vi "Motor Command.vi"(8 "error in (no error)":errorcluster, 11 "output cluster":T1) -> (0 "error out":errorcluster)   [LabVIEW 2016]
uses:
  Que Cluster TD.ctl
  Que Attributes TD.ctl
  Que enum td.ctl
  <vilib>/addons/zeromq/socket_type.ctl
  <vilib>/addons/zeromq/socket_options.ctl
  <vilib>/addons/zeromq/zeromq.lvlib
  <vilib>/addons/zeromq/zmq_context.lvclass
  <vilib>/addons/zeromq/zmq_socket.lvclass
panel:
  out "data":string
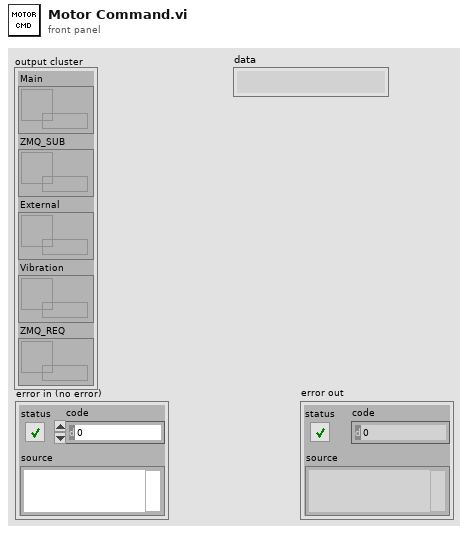
[diagram p1: front panel]
types:
  T1 = typedef "Que Cluster TD.ctl" = cluster{"Main":refnum<queue>, "ZMQ_SUB":refnum<queue>, "External":refnum<queue>, "Vibration":refnum<queue>, "ZMQ_REQ":refnum<queue>}
  T2 = typedef "zeromq.lvlib/socket_options.ctl" = enum8{"NONE", "ZMQ_HWM", "<2>", "ZMQ_SWAP", "ZMQ_AFFINITY", "ZMQ_IDENTITY", "ZMQ_SUBSCRIBE", "ZMQ_UNSUBSCRIBE", "ZMQ_RATE", "ZMQ_RECOVERY_IVL", "ZMQ_MCAST_LOOP", "ZMQ_SNDBUF", "ZMQ_RCVBUF", "ZMQ_RCVMORE", "ZMQ_FD", "ZMQ_EVENTS", "ZMQ_TYPE", "ZMQ_LINGER", "ZMQ_RECONNECT_IVL", "ZMQ_BACKLOG", "ZMQ_RECOVERY_IVL_MSEC", "ZMQ_RECONNECT_IVL_MAX", "ZMQ_MAXMSGSIZE", "ZMQ_SNDHWM", "ZMQ_RCVHWM", "ZMQ_MULTICAST_HOPS", "<26>", "ZMQ_RCVTIMEO", "ZMQ_SNDTIMEO", "<29>", "<30>", "ZMQ_IPV4ONLY", "ZMQ_LAST_ENDPOINT", "ZMQ_ROUTER_MANDATORY", "ZMQ_TCP_KEEPALIVE", "ZMQ_TCP_KEEPALIVE_CNT", "ZMQ_TCP_KEEPALIVE_IDLE", "ZMQ_TCP_KEEPALIVE_INTVL", "ZMQ_TCP_ACCEPT_FILTER", "ZMQ_DELAY_ATTACH_ON_CONNECT", "ZMQ_XPUB_VERBOSE"}
  T3 = typedef "zeromq.lvlib/socket_type.ctl" = enum8{"ZMQ_PAIR", "ZMQ_PUB", "ZMQ_SUB", "ZMQ_REQ", "ZMQ_REP", "ZMQ_DEALER", "ZMQ_ROUTER", "ZMQ_PULL", "ZMQ_PUSH", "ZMQ_XPUB", "ZMQ_XSUB"}
  T4 = typedef "Que Attributes TD.ctl" = cluster{"Que States":T5, "String":string, "Boolean":bool, "Double":dbl, "U16":u16}
  T5 = typedef "Que enum td.ctl" = enum16{"Stop", "Start", "Update D_HW", "Initialize", "Exit", "Read", "Write", "Plot", "Log", "Stop Log", "Start Log", "Wait"}
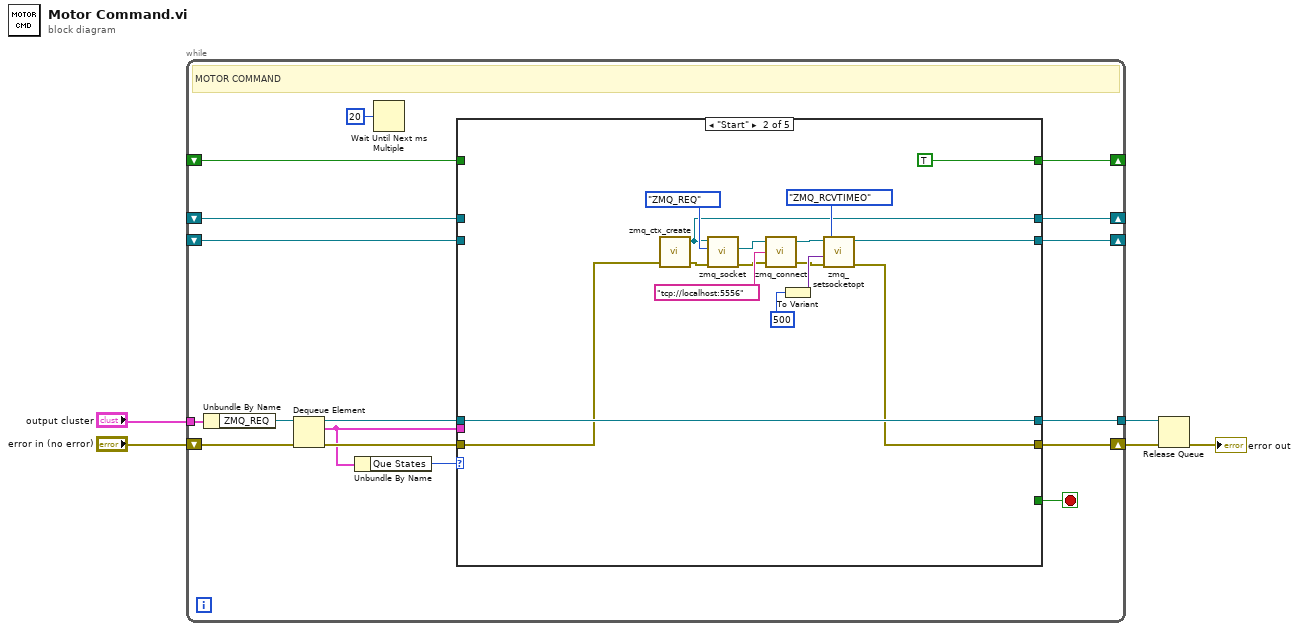
[diagram p0: block diagram]
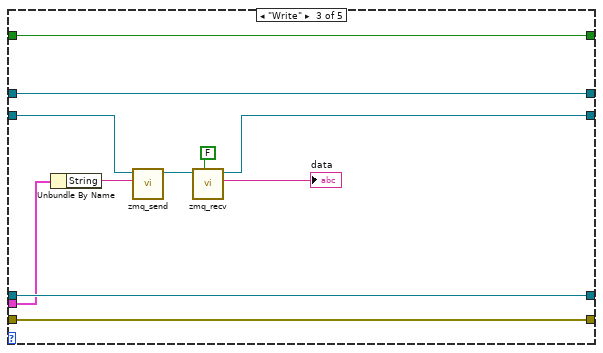
[diagram p3: hidden frame]
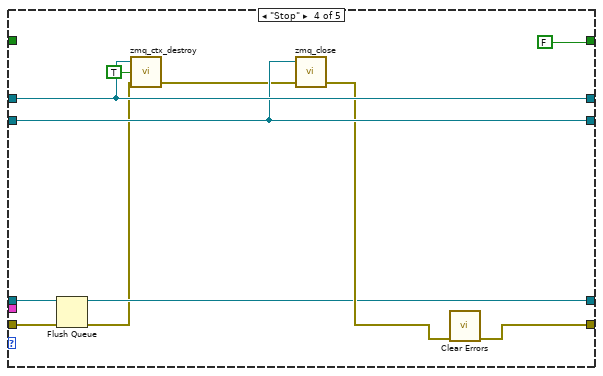
[diagram p4: hidden frame]
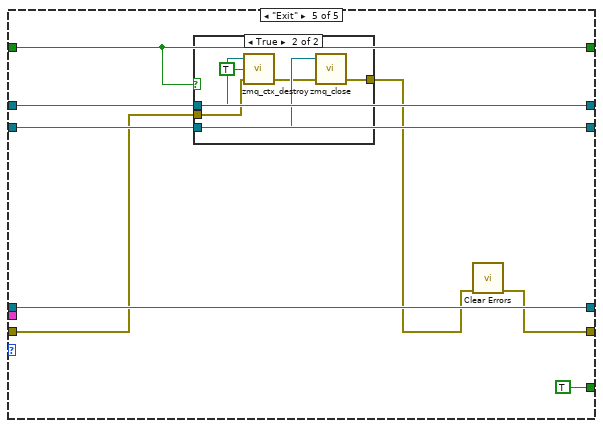
[diagram p5: hidden frame]
diagram:
  n1 = while {
    tunnel: "output cluster" -> [w22]
    tunnel: [w17] -> w4
    shift-right: [w16] -> w5
    shift-left: "error in (no error)" -> [w20]
    shift-right: [w12] -> _
    shift-left: _ -> [w11]
    shift-right: [w9] -> _
    shift-left: _ -> [w8]
    shift-right: [w7] -> _
    shift-left: _ -> [w6]
    stop <- w13 stop-if-true
    # "MOTOR COMMAND"
    n2 = Unbundle By Name(w22) -> ("ZMQ_REQ"=w21:refnum<queue>)
    n3 = Dequeue Element(queue=w21, error in (no error)=w20) -> (queue out=w18:refnum<queue>, element=w10:T4, error out=w19:errorcluster)  [unwired: 1 in, 1 out]
    n4 = Unbundle By Name(w10) -> ("Que States"=w15:T5)
    n5 = Wait Until Next ms Multiple(millisecond multiple=u32 20) -> ()  [unwired: 1 out]
    n6 = case shown="\"Start\"" w15 {
      tunnel: w19 -> [w26 w42 w47 w57 w68]
      tunnel: w18 -> [w27 w43 w54 w59 w73]
      tunnel: [w27 w43 w54 w58 w73] -> w17
      tunnel: [w26 w41 w47 w61 w66] -> w16
      tunnel: [_ _ _ _ TRUE] -> w13
      tunnel: [w25 w40 w50 w64 w70] -> w12
      tunnel: w11 -> [w25 _ w51 w64 w70]
      tunnel: w10 -> [_ _ w49 _ _]
      tunnel: [w24 w29 w45 w65 w71] -> w9
      tunnel: w8 -> [w24 _ w45 w65 w71]
      tunnel: [w23 TRUE w44 FALSE w69] -> w7
      tunnel: w6 -> [w23 _ w44 _ w69]
      frame "Initialize", Default {
      }
      frame "Start" {
        n7 = call <vilib>:"zmq_ctx_create.vi"("error in"=w42) -> ("error out"=w33:errorcluster, "context out"=w29:refnum<class "zmq_context.lvclass">)  [unwired: 3 in]
        n8 = call <vilib>:"zmq_socket.vi"("error in"=w33, "socket type"=socket_type."ZMQ_REQ", "context in"=w29) -> ("error out"=w30:errorcluster, "socket out"=w31:refnum<class "zmq_socket.lvclass">)  [unwired: 2 in, 1 out]
        n9 = call <vilib>:"zmq_connect.vi"("error in"=w30, "endpoint"="tcp://localhost:5556", "socket in"=w31) -> ("error out"=w36:errorcluster, "socket out"=w35:refnum<class "zmq_socket.lvclass">)  [unwired: 1 in]
        n10 = To Variant(anything=500) -> (Variant=w39:variant)
        n11 = call <vilib>:"zmq_setsocketopt.vi"("error in"=w36, "value"=w39, "option"=socket_options."ZMQ_RCVTIMEO", "socket in"=w35) -> ("error out"=w41:errorcluster, "socket out"=w40:refnum<class "zmq_socket.lvclass">)  [unwired: 2 in]
      }
      frame "Write" {
        n12 = Unbundle By Name(w49) -> ("String"=w48:string)
        n13 = call <vilib>:"zmq_send.vi"("data"=w48, "socket in"=w51) -> ("socket out"=w52:refnum<class "zmq_socket.lvclass">)  [unwired: 5 in, 1 out]
        n14 = call <vilib>:"zmq_recv.vi"("no block? (F)"=FALSE, "socket in"=w52) -> ("data"=→"data":string, "socket out"=w50:refnum<class "zmq_socket.lvclass">)  [unwired: 3 in, 3 out]
      }
      frame "Stop" {
        n15 = Flush Queue(queue=w59, error in (no error)=w57) -> (queue out=w58:refnum<queue>, error out=w56:errorcluster)  [unwired: 1 out]
        n16 = call <vilib>:"zmq_ctx_destroy.vi"("error in"=w56, "reap? (F)"=TRUE, "context in"=w65) -> ("error out"=w63:errorcluster)  [unwired: 2 in]
        n17 = call <vilib>:"zmq_close.vi"("error in"=w63, "socket"=w64) -> ("error out"=w62:errorcluster)  [unwired: 3 in]
        n18 = call <vilib>:"Clear Errors.vi"("error in (no error)"=w62) -> ("error out"=w61:errorcluster)  [unwired: 5 in, 1 out]
      }
      frame "Exit" {
        n19 = case shown="True" w69 {
          tunnel: w71 -> [_ w80]
          tunnel: w70 -> [_ w79]
          tunnel: w68 -> [w74 w78]
          tunnel: [w74 w76] -> w67
          frame False {
          }
          frame True {
            n20 = call <vilib>:"zmq_ctx_destroy.vi"("error in"=w78, "reap? (F)"=TRUE, "context in"=w80) -> ("error out"=w77:errorcluster)  [unwired: 2 in]
            n21 = call <vilib>:"zmq_close.vi"("error in"=w77, "socket"=w79) -> ("error out"=w76:errorcluster)  [unwired: 3 in]
          }
        }
        n22 = call <vilib>:"Clear Errors.vi"("error in (no error)"=w67) -> ("error out"=w66:errorcluster)  [unwired: 5 in, 1 out]
      }
    }
  }
  n23 = Release Queue(queue=w4, error in (no error)=w5) -> (error out=→"error out":errorcluster)  [unwired: 1 in, 2 out]
